vi "load.vi"(10 "名称或相对路径":path, 11 "基路径":path) -> (3 "数组":string[][](array[string]))   [LabVIEW 2022 SP3]
uses:
  <vilib>/Utility/file.llb/Read Delimited Spreadsheet (string).vi
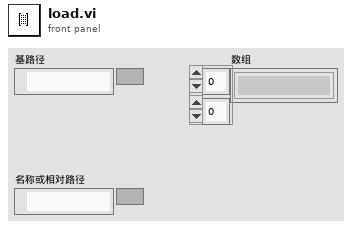
[diagram p1: front panel]
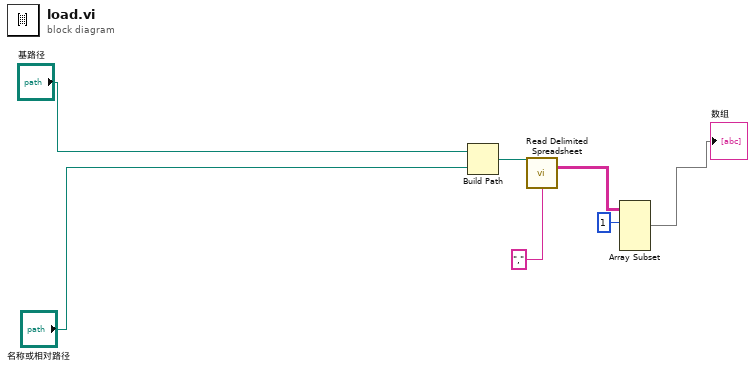
[diagram p0: block diagram]
diagram:
  n1 = Build Path(base path="基路径", name or relative path="名称或相对路径") -> (appended path=w3:path)
  n2 = call-poly <vilib>:"Read Delimited Spreadsheet.vi"("file path (dialog if empty)"=w3, "delimiter (\\t)"="," ("delimiter (\\t)")) -> ("all rows"=w2:string[][])  [unwired: 8 in, 5 out]
  n3 = Array Subset(array=w2, index (row)=1 ("索引")) -> (→"数组":string[][])  [unwired: 3 in]
